vi "configure.vi"(8 "error in (no error)":errorcluster, 9 "Value":i32, 10 "ILC":refnum<class "ILC.lvclass">, 11 "IConfigureILCStrategy in":refnum<class "ConfigureILCROTStrategy.lvclass">) -> (0 "error out":errorcluster, 2 "ILC 2":refnum<class "ILC.lvclass">, 3 "IConfigureILCStrategy out":refnum<class "ConfigureILCROTStrategy.lvclass">)   [LabVIEW 2016, in "ConfigureILCROTStrategy.lvclass"]
uses:
  ConfigureILCROTStrategy.lvclass
  Common_ILC/ILC/ILC.lvclass
  Common_ILC/ILC/ILC.lvclass/ILC.ctl
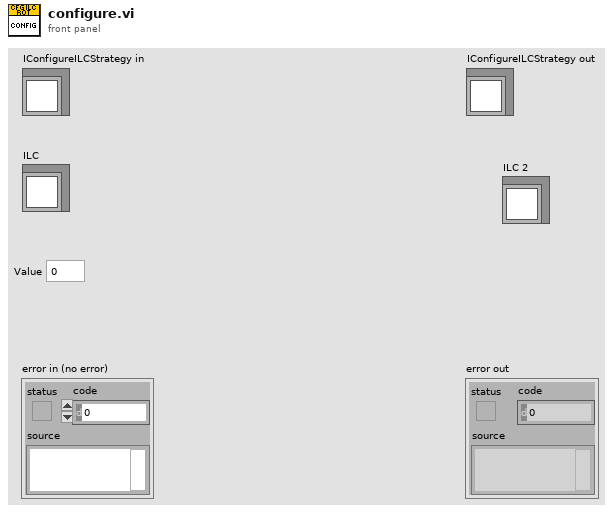
[diagram p1: front panel]
types:
  T1 = typedef "ILCCommon.lvlib/ILCTypedefs.lvlib/Outputs.ctl" = cluster{"Step & Direction":i16, "Blower RPM":u8, "PWM (SSR)":u8, "Ch1":u16, "Ch2":u16, "Ch3":u16, "Ch4":u16}
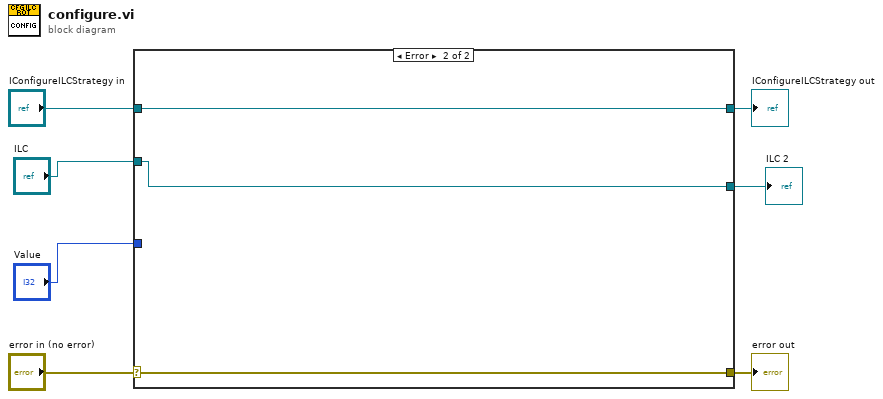
[diagram p0: block diagram]
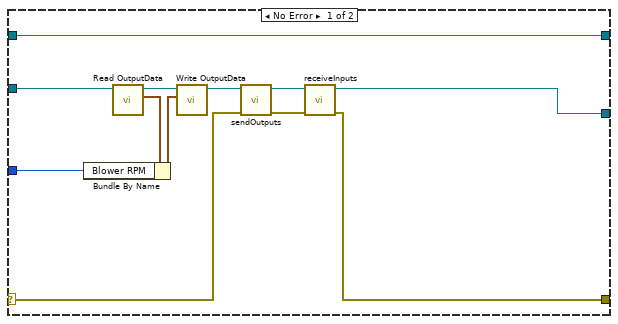
[diagram p2: hidden frame]
diagram:
  n1 = case shown="Error" "error in (no error)" {
    selector: "error in (no error)" -> [w11 w22]
    tunnel: [w9 w22] -> w6
    tunnel: [w19 w21] -> w4
    tunnel: "IConfigureILCStrategy in" -> [w19 w21]
    tunnel: "ILC" -> [w18 w20]
    tunnel: "Value" -> [w16 _]
    tunnel: [w8 w20] -> w1
    frame No Error {
      n2 = call "Read OutputData.vi"("ILC in"=w18) -> ("OutputData"=w17:T1, "ILC out"=w14:refnum<class "ILC.lvclass">)  [unwired: 9 in]
      n3 = Bundle By Name(cluster=w17, "Blower RPM"=w16) -> (w15:T1)
      n4 = call "Write OutputData.vi"("OutputData"=w15, "ILC in"=w14) -> ("ILC out"=w13:refnum<class "ILC.lvclass">)  [unwired: 9 in]
      n5 = call "sendOutputs.vi"("error in (no error)"=w11, "ILC in"=w13) -> ("error out"=w10:errorcluster, "ILC out"=w12:refnum<class "ILC.lvclass">)  [unwired: 8 in]
      n6 = call "receiveInputs.vi"("error in (no error)"=w10, "ILC in"=w12) -> ("error out"=w9:errorcluster, "ILC out"=w8:refnum<class "ILC.lvclass">)  [unwired: 6 in, 2 out]
    }
    frame Error {
    }
  }
  "error out" <- w6
  "IConfigureILCStrategy out" <- w4
  "ILC 2" <- w1
